vi "FindAndTrackFaces.vi"(8 "error in (no error)":errorcluster, 10 "Image in":T1, 11 "Object Tracking Session In":T2) -> (0 "error out":errorcluster, 1 "Face Images":T1[](array[typedef]), 2 "Image out":T1(plugin-control), 3 "Object Tracking Session Out":T2)   [LabVIEW 2019]
uses:
  <vilib>/vision/Image Controls.llb/IMAQ Image.ctl
  <vilib>/vision/Tracking.llb/IMAQ Object Tracking Session.ctl
  <vilib>/vision/NI_Vision_Development_Module.lvlib
panel:
  out "size(s)":i32
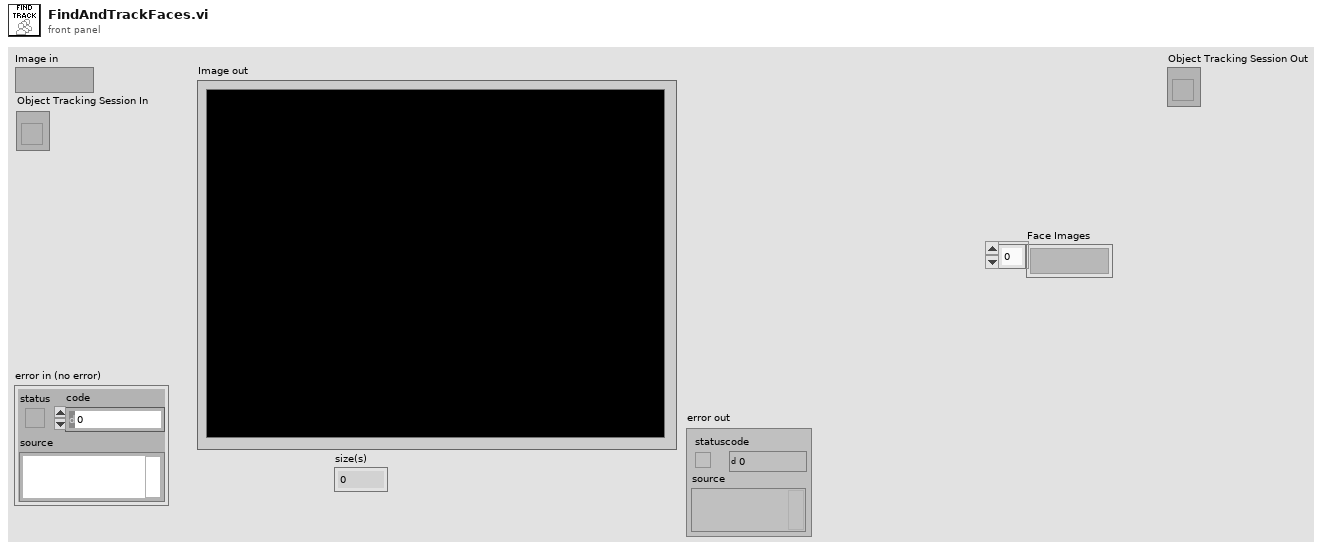
[diagram p1: front panel]
types:
  T1 = typedef "IMAQ Image.ctl" = refnum<image>
  T2 = typedef "IMAQ Object Tracking Session.ctl" = refnum<k20>
  T3 = typedef "IMAQ Rectangle" = cluster{"Left":i32, "Top":i32, "Right":i32, "Bottom":i32, "Rotation":dbl}
  T4 = cluster{"Label":string, "Score":i32, "Angle":dbl, "Location":cluster{"X":dbl, "Y":dbl}, "Bounding Box":cluster{"X":dbl, "Y":dbl}[], "Object Found?":bool}[]
  T5 = typedef "Image Type" = u32
  T6 = typedef "ROI Descriptor" = cluster{"Global Rectangle":i32[], "Contours":cluster{"ID":enum32{"External", "Internal"}, "Type":u32, "Coordinates":i32[]}[]}
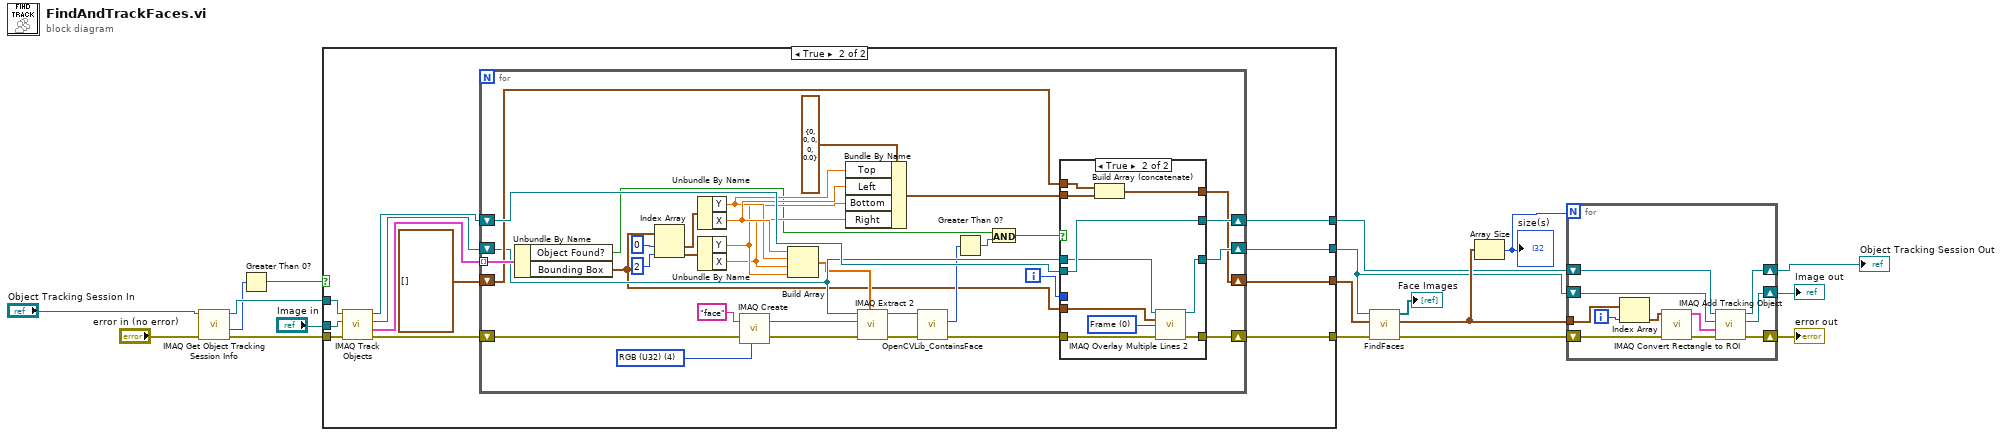
[diagram p0: block diagram]
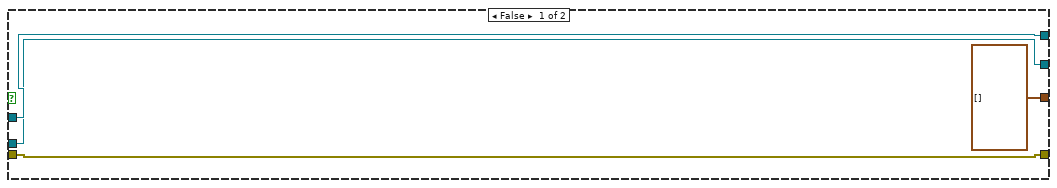
[diagram p2: hidden frame]
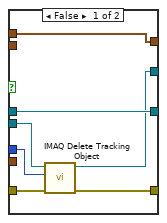
[diagram p3: hidden frame]
diagram:
  n1 = call "IMAQ Get Object Tracking Session Info"("error in (no error)"="error in (no error)", "Object Tracking Session In"="Object Tracking Session In") -> ("error out"=w8:errorcluster, "Number of Objects"=w9:i32, "Object Tracking Session Out"=w11:T2)  [unwired: 6 in, 1 out]
  n2 = Greater Than 0?(x=w9) -> (x > 0?=w10:bool)
  n3 = case shown="True" w10 {
    tunnel: "Image in" -> [w21 w32]
    tunnel: w11 -> [w22 w31]
    tunnel: w8 -> [w20 w30]
    tunnel: [w20 w29] -> w17
    tunnel: [w21 w28] -> w7
    tunnel: [w22 w25] -> w14
    tunnel: [T3[] [] w24] -> w6
    frame False {
    }
    frame True {
      n4 = call "IMAQ Track Objects"("error in (no error)"=w30, "Image"=w32, "Object Tracking Session In"=w31) -> ("error out"=w33:errorcluster, "Objects (pixel)"=w27:T4, "Image (duplicate)"=w34:T1, "Object Tracking Session Out"=w26:T2)  [unwired: 1 in, 4 out]
      n5 = for {
        shift-right: [w65] -> w28
        shift-left: w34 -> [w48]
        shift-right: [w67] -> w29
        shift-left: w33 -> [w45]
        tunnel: w27 -> [w66] mode=indexing
        shift-right: [w62] -> w25
        shift-left: w26 -> [w63]
        shift-right: [w38] -> w24
        shift-left: T3[] [] -> [w61]
        i -> [w64]
        w36 = T5 4 items=["Grayscale (U8)", "Grayscale (I16)", "Grayscale (SGL)", "Complex (CSG)", "RGB (U32)", "HSL (U32)", "RGB (U64)", "Grayscale (U16)"] ("Image Type")
        n6 = Unbundle By Name(w66) -> ("Object Found?"=w42:bool, "Bounding Box"=w35:cluster{"X":dbl, "Y":dbl}[])
        n7 = Index Array(array=w35, index #1=0 ("index"), index #2=2 ("index")) -> (element #1=w57:cluster{"X":dbl, "Y":dbl}, element #2=w56:cluster{"X":dbl, "Y":dbl})
        n8 = Unbundle By Name(w57) -> ("Y"=w54:dbl, "X"=w55:dbl)
        n9 = Unbundle By Name(w56) -> ("Y"=w53:dbl, "X"=w52:dbl)
        n10 = call "IMAQ Create"("Image Name"="face", "Image Type"=w36, "error in (no error)"=w45) -> ("New Image"=w50:T1, "error out"=w46:errorcluster)  [unwired: 2 in]
        n11 = Build Array(w55, w54, w52, w53) -> (w47:dbl[])
        n12 = Bundle By Name(cluster=T3 {"Left"=0, "Top"=0, "Right"=0, "Bottom"=0, "Rotation"=0.0} ("Rectangle"), "Top"=w54, "Left"=w55, "Bottom"=w53, "Right"=w52) -> (w40:T3)
        n13 = call "IMAQ Extract 2"("Optional Rectangle"=w47, "error in (no error)"=w46, "Image Dst"=w50, "Image Src"=w48) -> ("error out"=w37:errorcluster, "Image Dst Out"=w49:T1)  [unwired: 6 in]
        n14 = call "OpenCVLib_ContainsFace.vi"("error in (no error)"=w37, "Image Src"=w49) -> ("error out"=w39:errorcluster, "containsFace"=w44:i8)  [unwired: 7 in, 1 out]
        n15 = Greater Than 0?(x=w44) -> (x > 0?=w43:bool)
        n16 = And(x=w42, y=w43) -> (x .and. y?=w41:bool)
        n17 = case shown="True" w41 {
          tunnel: w48 -> [w74 w78]
          tunnel: [w74 w80] -> w65
          tunnel: w39 -> [w72 w81]
          tunnel: [w71 w79] -> w67
          tunnel: w64 -> [w73 _]
          tunnel: w63 -> [w70 w84]
          tunnel: [w69 w84] -> w62
          tunnel: [w68 w83] -> w38
          tunnel: w61 -> [w68 w82]
          tunnel: w40 -> [_ w77]
          tunnel: w35 -> [_ w76]
          frame False {
            n18 = call "IMAQ Delete Tracking Object"("error in (no error)"=w72, "Object Index"=w73, "Object Tracking Session In"=w70) -> ("error out"=w71:errorcluster, "Object Tracking Session Out"=w69:T2)  [unwired: 7 in]
          }
          frame True {
            w75 = u32 0 items=["Frame", "Fill"] ("Drawing Mode (Frame)")
            n19 = Build Array (concatenate)(w82, w77) -> (w83:T3[])
            n20 = call "IMAQ Overlay Multiple Lines 2"("Image"=w78, "Line End Points"=w76, "Drawing Mode (Frame)"=w75, "error in (no error)"=w81) -> ("Image Out"=w80:T1, "error out"=w79:errorcluster)  [unwired: 10 in]
          }
        }
      }
    }
  }
  n21 = call "FindFaces.vi"("error in"=w17, "Faces In"=w6, "Image In"=w7) -> ("error out"=w13:errorcluster, "Faces"=w15:T3[], "Array"=→"Face Images":T1[])  [unwired: 6 in]
  n22 = Array Size(array=w15) -> (size(s)=w16:i32)
  "size(s)" <- w16
  n23 = for {
    N: w16 -> [_]
    tunnel: w15 -> [w88]
    shift-right: [w93] -> w4
    shift-left: w14 -> [w94]
    shift-right: [w89] -> w12
    shift-left: w13 -> [w90]
    shift-right: [w85] -> w2
    shift-left: w7 -> [w95]
    i -> [w86]
    n24 = Index Array(array=w88, index=w86) -> (element=w87:T3)
    n25 = call "IMAQ Convert Rectangle to ROI"("error in (no error)"=w90, "Rectangle"=w87) -> ("error out"=w91:errorcluster, "ROI Descriptor"=w92:T6)  [unwired: 7 in]
    n26 = call "IMAQ Add Tracking Object"("error in (no error)"=w91, "ROI Descriptor"=w92, "Image"=w95, "Object Tracking Session In"=w94) -> ("error out"=w89:errorcluster, "Image (duplicate)"=w85:T1, "Object Tracking Session Out"=w93:T2)  [unwired: 1 in, 4 out]
  }
  "Image out" <- w2
  "Object Tracking Session Out" <- w4
  "error out" <- w12
